vi "clustering.vi"() -> ()   [LabVIEW 2013]
panel:
  in  "sub patterns out":string[](array[string])
  in  "subpatterns out":string[](array[string])
  in  "Sub patterns":string[](array[string])
  in  "top":string[](array[string])=["0 4 0 4 0 4 0 4 0 -2 3 0 3 0 4 0\r\n", "-4 -1\r\n", "-2 0 1 0 -4 4\r\n", "0 4\r\n", "-2 2 0 -1 -4 1 0 3 0\r\n", "-1 0 -1 2\r\n", "0 -1 1 0 4 0 3 -2 0 -2 3 -2 0 4 0 -2 2\r\n", "2 -1 0 4\r\n", "0 4 0 2 0 -2 0\r\n", "1 -1 0 3 0 -4 4 -4 0\r\n", "2 -1 0 3 -2 0 -3 0 3 0 -3 0\r\n", "0 4 0 4 -4 1 -1 0 -3 0 1 -4 1 0 4 0 -4 0 -4 4 -4 1\r\n", "0 -4 1 0 -4 4\r\n", "0 4 0 -2 2 -2 2 -2 2\r\n", "-2 2 -1 0 4 0 2 0 4 0 2 -2 0 4\r\n", "1 0 -1 0 -1 0 1 -1\r\n", "-2 2 -2 3\r\n", "1 0 -1 0 -1 2 0 2 -2 0 -4 0\r\n", "-2 2 0 3 -2 2\r\n", "0\r\n", "1 -1 0 3\r\n", "0 4 0\r\n", "-2 0 1 -4 0 -3 0\r\n", "1 0 -1 2 -1 1 -4\r\n", "0 4\r\n", "-2 0 -1 1\r\n", "0 3 0 3 0 3 -2\r\n", "-4 0 -4 4\r\n", "0 4 0 -4 0 -4\r\n", "-2 2 0 4 -4 0 2 -2\r\n"]
  out "bottom":string[](array[string])
  in  "MOM set 2 bottom CJ vs MOM":string[](array[string])=["-2 0", "0 4 0 3 0 4 0 2 0", "0 3 -2 0 4 0 2 0 4 0 2", "0 2 0 1 0", "0 4 -3 0 -2 0", "0 3 0 4 0 3 0 3 0", "0 3 0 3 0", "0 1 0 -3 3 -3 0 4 0", "0", "0 -3 4 0 3 -2 3 0 1 0 4 0", "0", "0 2 0 3 0 -2 0 -2 0 3 0 1 0", "0 3 0 -3 4 0", "0 3 -2 2 0 3 0 3 0", "0 3 0 3", "0", "-1 0 1", "0 4 0 1", "0 2 0 4 0", "0 1 0 4 0 -4 1 0 3", "0 3", "0 -3 4 0 3 0 3 -2 0 1 0 3 0 3 0", "0 2 0 3", "0 3 0 3 0", "0 1 0 4 0 -2 0 3 0 -4 0 4 0 -4 1 0 3 0 3 0 1", "0 2 0 -3 4 0", "0 3", "0 3", "0 1 0 4", "0", "0 3 0 1 0 3 0 4"]
  in  "WF set 2 bottom CJ vs WF":string[](array[string])=["-2 2 0 4 0 -4 0 3 0", "0 1", "0 3 0 -2 2 -2 3 0 3 -3 0 1 0 3 0 4 0 -2 3", "-2 2 0 3", "0 1 0 4 0 4 -4 1 -1 2 0 3 -3 0 -2", "0 4 -3 0", "0 3", "0 1 0 3 0 2 0 -3 0 4 0 3 0 -2 0 -3 0 -4 0 3 0", "-2 2 -2 3 -3 0 -4 1", "0 4 0", "0 4 0 1 0 4 0 3", "-2 0 2 0 4 0 3", "0 4 0 3 0 4 0 4 0 3 0 3", "-2 2 0 4 0 3 0 2 0 3 -2", "0 3 0 3 0 3 0 3 0 3 0 3 0 4 0 1 0 -2 3 0 3", "0 2 0 -3 4", "1 0 3 0 2", "0 1 0", "-2 2 0 -2 3", "0 1 0 4 0 3 -2 0 -3 0 -3 4 0 1 0 2 0 3 0 1 0 3 0 3 0 4 0 -4 0 3 0 -3 0 2", "0 4 0 1", "0 3 0 4 0 1 0 -2 0", "-2 2 0", "0", "0 2 0", "0 1 0 3", "-2 2 0 -4 4 0 3 0 4 0 -4 0 3 0", "0 2 0 1 0 4 0 1 0 4 0 4 0 3 0", "0 1 0 4 -3 0 2 0 4 0 4 0 -4 0 4 0 1 0 3 0", "0 2 0 3 0"]
  in  "CJ set 2 top CJ vs WF":string[](array[string])=["0 -4 4 -4 0 3 0 4", "0", "-4 1 0 -4 1 0 2 0 -4 0 3 0 1 0 -4 4", "0 -4", "0 2 0 4 -4 0 -1 1 0 -3 0", "-4 0 1", "0 -4 0", "0 -3 0 2 -2 2 0 1 0 1 0 -4 4 -4 1 0 3 0 1", "0 1 0 2", "0 4 -4 1 -4 1 0 1 0 3 0 2", "-4 0 -2 0 2 0 3 0 1", "0 -3 0 4 0 -4 1 -4 1 0", "0 3 0 1 0 3 0 3 0 -4 4 0", "0 4 0 -1 0 3 0 -4 0 1 0 -4 4 -4", "0 -1 1 0 4 -3 4 0 2 0 -4 4 0 -4 4 -4 0 4 0 4 0 1 -1 0 -3 0 -2 3 -2 3 0 3 0 3 0 1 0 -4 0", "0 1 0", "0 3 0 1 0 1 0 4", "0 -3 0 2 -1", "0 4", "0 -3 0 3 0 -4 4 -4 0 -4 4 -4 1 0 2 0 3 0 3 0 4 0 -2 0 1 0 4 0 2 -1 0 3 0 3 0 1", "1 0 4 -4 1 0 2", "0 3 0 2 0 3 0 4 -4 1", "0 4 0 -1 0", "0", "0 4", "-3 0 2 0", "0 -3 0 -3 0 -4 4 0 3 0 2 -2 0 4", "-4 0 4 0 3 0 4 0 3 0 1 0 4", "0 3 0 -4 4 -3 0 4 0 3 0 2 0 2 0 4 0 -4 4 -4 0", "0 1 0 -4 4 -4 0"]
  in  "CJ set 1 bottom CJ vs WF":string[](array[string])=["0 2 0 3 0", "-4 0 4 0 4 0 -4 0 2 0 4", "-1 0 3 0 3 -3 0 4 0 -4 0 3 0", "0 2 0 4 0 3 0 1 0", "0 4 0", "-4 0 3 0 1 0 3", "0 1 0 3 0 1 0 4 0", "0 4 0 3 0 2 0 4 -4 1 0 3 0 3 0 2 0", "0 4", "0 3 0 3 0 3 0 -3 4 0 4 0 2", "-4 1 0 4 -3 0 3 0 4 0 2 0", "0 1 0 4 -3 0 -2 0 -2 2 0 3 0 3 0 -2 2 0 4", "0 1 0 -2 -3 4", "-1 0 4 -3 0 -2 0 1 0 1 0", "0 3", "0 2 -1 0 4 -4 1 0 3 0", "0 1 0 3 0 4 0 3 -2 0", "0 3 0 -4", "0", "0 1 0 -2 0 3 0 1 0 3 0 3 -3 0 4 0", "0 -3 4 0 3 -2 0 -2 2 0 4 0 3 -3 0 1 0 3 0 4 0", "0 3 0 -4 0 2", "0 -4 0 -2 0 -1 0 3 0 1 0 -3 0 3 0 4 0", "-4 0 1 0", "0 4 0", "0 2 0", "0 2 0", "0 3 0 1 0 3 0 -4 0 2 0 -4 0 2 0 -3 4 0 -2 0 3 0 -2 0 -1 1", "0 2 0 4 0 3 -3 4 0 2 0 3 0 1 0 3 0 -4 0 4 0 2 0 4 0 1 0 1 0 2 0 4 -4 1 0 2", "0 1 0 2 0 3 -3 0 1", "-4 0", "0 4 0 -1 0 4", "0 4 0 2 0 4 0 4 -4 0 -2 2 0 -4 4 0 3 0 2 0 2 0 3 0 1 0 2", "0 4", "-1 0 2 0 1"]
  in  "WF set 1 top CJ vs WF":string[](array[string])=["-1 0 1 0", "0 3 0 3 0 3 0 2 0 3 0", "1 0 1 0 4 0 3 0 -2 3 -2 0 3", "0 3 0 1 0 2 0", "0 2 0 4", "0 4 0 1 -1 0 -3", "1 -1 0 4 0 4 0 2 -2 0 -4 0 -3 3 -2 3 0", "2 -1 0 1 0 3 0 3 0 4 0 -4 4 -4 -1 0 3", "0 3", "1 0 2 0 3 0 4 0", "0 2 0 -3 4 0 -1 0 4 0 4 -4 0 2 -1 1 0 3 0", "0 3 -2 3 0 4 0 1 0 4 0 4 0 4 0 3", "2 0 3 0 -4 1 0", "0 1 0 1 -1 0 -1 3 -2 2 0 -3 0 1", "2 0", "0 1 0 3 0 3 0", "0 4 0 1 0 1 0 3 0 4 0 -4 4", "2 0 4 0 -1", "0 3", "0 4 0 1 0 4 -4 0 -3 0 -4 4 0 3 0 -1 1 -4 4", "0 1 0 -4 0 4 0 1 0 4 0 2 0 4 0 2 -2 0 3 0 4 0 3 0 4 0 4", "1 0 4 0 2 0", "2 0 4 0 1 -1 0 4 0 2 0 4 0 1 0 4 0 2", "0 4 0 3 0", "0 3 0 -2 3 0 1", "0 1 0 1 0 -1 0 3 -2 2 0", "2 0 3", "0 1 0 -1 0 2 0 4 0 3 0 1 -1 0 4 -4 0 -1 2 0 1 0 3 0 4 0 3 0 1 -1 0 3", "2 0 3 0 4 0 1 0 4 0 -4 0 3 0 4 0 4 0 2 0 4 0 3 0 3 0 3 -2 3 -3 0 3 0 3 0 -4 1", "1 0 3 0 -3 0 3 0 3 -2 2", "0 4", "2 0 3 0 2 0 -1 0 -3 0", "0 3 0 -4 0 3 0 3 0 3 0 3 0 1 0 3 0 3 0 4 -4 0 1 0 3 0 -3 0 -4 0 3 0 1", "0 -1 0 3", "0 2 0 3 0"]
  in  "CJ set 2 top CJ vs MOM":string[](array[string])=["0 2", "0 2 -1 0 -1 0 4 -4 0 1 0", "-4 1 0 -1 0 -4 4 -4 1 0 4 -4 0", "0 -3 0 2 0", "0 2 0 -4 1 0", "2 0 -2 2 0 -2 0 -4 4 -4 0 4", "0 3 0 -3 4 0 1 0 4", "0 2 0 2 0", "0 4 0", "0 -1 1 -1 0 -2 3 0 1 0 1 0 1 0 3 0", "-4 1 -4 1", "0 -1 0 -4 4 -4 1 -4 1 0 4 -4 1", "0 1 0 1 0 1 0", "0 2 0 -4 0 -1 0 4 -4 0", "-4 1 0 -4 4", "0 3 0 2", "3 0", "0 2 0 -2 0", "-3 0 4 -4 0 4 0", "0 3 0 -2 2 -1 0", "0 -1 0", "0 1 0 1 -4 1 0 4 0 2 0 4 0 3 0 4 -4 1 0 4", "0 4", "-4 1 0 -1 0 -1 0 -2", "-3 0 3 0 -2 0 2 0 4 0 -1 1 0 -2", "-3 0 1 0 1 0", "0 2 -1 0", "1 -4 1 0 4", "0 4 0", "0 2", "0 3 0 4 0 4 -4 0 2"]
  in  "CJ set 1 bottom CJ vs MOM":string[](array[string])=["0 4 -4 0 3 0 4 0", "-4 0 -4 0", "-1 0 3 0 4 0", "0 3", "-1 0 3 0 2 0 4", "-1 0 4 0 2 0 3 -3 0 1 0 2 0", "0 3 -3 0 4", "-1 0 1 0", "2 0 2 0 4 -4 1 0 3", "0 3 0 4 0 -3 0 -3 0 3 -3 0 -2 0 4 0 4 0 -4 0 -4 0 4", "0 -3 0 1 0 4", "0 1 0 -4 0 4 0 -2 0 2 0 4 0 -4 0 3 0 3 0", "-4 0", "0 4 0 -3 0", "-4 4 -4 1 0 -4 4 0 -3 0 -3", "0 -3 3 -3 0 2 0 4 -4 0 -3 3 -3 0", "0 2 0 4 -3 3", "0 -4", "0 2 0 -4 4 0 -2", "-4 1 0 4 0 3 0 3 -2 0 -4 0 1 0 -3 3 -3", "0 -4", "0 -3 0 -3 0 -4 0 -3 3 0", "-1 0 4 0 4 0 4", "0 -3 3 0 2 0 2 0", "0 4 -3 0 4 0 -2 0 4", "-4 0 -4 0 1 -4", "0 4 0 -3 4 0 4", "0 1 0", "0", "-1 0 3 0 3 -3 0 -3 0", "-3"]
  in  "MOM set 1 top CJ vs MOM":string[](array[string])=["2 -1 0 3 0 -2 0 3 0 3", "0 3 -2 2 -1", "1 0 4 0 4 0 2 0 2 0", "2 -1 0", "0 1 0 1 0", "2 0 -2 0 3 -2 0 4", "1 0 4 0 -2 3 -2", "2 0 -2 3", "-3 0 2 0 4 0 4", "-1 0 -1 0 2 0 1 0 4 -4 1 -1 2 -2 3 -2 0 -2 3 0 4 0 3 -2", "2 -1 0 3 -2", "-1 0 2 -2 3 -2 0 -1 0 2 -2 3 0", "0 2", "0 2 0 1", "0 -2 2 -2 3 -2 2 -2 0 1 0", "2 0 2 0 3 -2 2 0 -1 1 0 2", "-1 0 2 -1 0", "2 -2", "-1 0 -1 1 -1 0 -3 0 -2 3 -2", "0 2 -1 0 4 0 -2", "0", "-1 0 2 -1 0 2 -2 3 -2 3 -2 0 2", "2 -2 2 0 2", "-1 0 4 0 3 -2 2 -1 0 -2 3 0 -1", "2 -1 1 -1 0 3 -2 3 0 -2 2 0 -2 3 -2 0 1 0 4 0 2", "0 -2 0 2 -2", "-1 0 2 0 2 0 -2 3", "2 0", "0 -1 0 -2 0 -2", "-1 0", "-1"]
  in  "HY set 2 bottom CJ vs HY":string[](array[string])=["0 2 0", "0 4", "0 1 0", "0", "0 3 0 3 0 -1 0 4 0 -3", "0 4 0 -2 0 1 0 4 0 4 0 1 0 3 -3 0", "0 1 0 2", "0 2 0 4", "1 0 1 0 3 0 3 0 3", "0 1 0 4 0 3 0 -2 0", "-1 0 2 0 3 0 -4 1 0 4 0", "0 2 0 -4 0 -4 4 0", "0 1 -1 2", "0 4 0 2 0 3 0 -2 0 -4", "0", "0 1", "0 4 0 -1 1 0", "0", "0", "0 1 0 4 0 -4 0 4 0 -4 0", "0 3 0 -2 0 3 0 2", "0 1", "0 2", "0", "-1 0 4 0 -3 0 -2 0 -2 0 1 0 -4 0 4", "2 -1", "0 -1 0 4 0 4 -4 0 -1 2", "0 -2 0", "0 3 0", "-1 0 -3 0", "0 2 0 1", "0 1 0 1", "0 4 0 2 0 -4 1 2 0 4 0 4 0 4", "0"]
  in  "CJ set 2 top CJ vs HY":string[](array[string])=["0 -1 1", "0 1 0", "0 3 0 4 0 -1 0", "0 4 -4 0 1", "0 4 0 1 -1 0 -3 0 4 0 -1 0 4", "0 -3 0 2 0 4 0 2 -1 0 4 -4", "0 1", "0 4 0 1 0 -1 0", "0 2 -1 0 -4 4 0 1", "0 2 0 4 -4 1", "4 -4 0 4 0 2 0 3 0 4", "0 4 0 2 0 4", "0 -1 1 -1", "0 -4 0 -4 4 0 4 0 4 -4 1 0 3", "0 -1", "0 2 0 2", "0 3 0 1 0", "0 2 0", "0", "0 4 -4 1 -4 0 3 -2 0 4 0 4 0", "0 2 0 4 -4 1 0 1", "0", "0", "0", "0 2 0 -1 0 4 -4 1 0 1 0 1 0 4 0 4 0 2", "0 -1", "-4 1 0 4 0 -2 0 3 0 -1 1", "0 -2 0 -4 0 4 -3 0", "0 -1 1 0", "4 0", "0 4 0", "0", "0 -4 0 4 0 2 -1 1 0 4 0 -3 0 -4 0 2 0 3 0 2 0", "0"]
  in  "CJ set 1 bottom CJ vs HY":string[](array[string])=["2 0 3 0 3 0 4 0 4 0 3", "0", "0 4 -3 0 3 0", "-1 0 4 1 0 3", "-4", "0 3 0 2 0", "0 1", "0 -3 3 0 3 -3 0 4 0 1 0 3 0 1", "-1 0 -1 0", "-4 0 -4 0 4 -4 0", "-1 0 4 0 2 0 3 0", "-1 0 1 0 3 -3 0 1 0", "0 2 0 3 0 2 0 4 0 4 0 2 0 3 0 2", "0 3", "1 -4 0", "0 -1 0 1 -4 4 0 3 0 4 0 2 0", "0 4 0 -2 2 0", "0 4", "0 1 0 4 0 3 0 3", "0 1 0", "0 2 0", "-1 0 4", "-4 0 -2 3", "0 3 0 1 0", "-1 0 1 -1", "0 2 0 3 0", "0 4 0", "-4 0 -4 0 4 0", "0 3 0", "0 3", "0 1 0"]
  in  "HY set 1 top CJ vs HY":string[](array[string])=["0 4 0 4 0 3 0 -2 3 0 4 0", "1", "2 -2 0 4", "1 0 4", "0", "-2 0 1 -4 1 0 3", "1 0", "0 -1 1 0 -4 0 3 0 3 0 4 0 -2 2", "2 0 4", "0 2 0 -2 0", "1 -1 0 3 0 4 -4 4 0", "0 3 2 0 -3 0 3 0 4", "0 -4 4 0 1 0 -3 0 1 0 4 0 -4 4 -4", "1 0 -4 4", "-3 0 4 0 2", "-2 2 0 4 0 2 0 4 0 2 0 -4 0", "1 0 -1 0 -1 0 1", "2 0 3", "1 0 2 0 3 0 2 0 -4 0", "-2 2 0 3 -2", "0", "1 -1 0 3", "0", "-2 0 1 0", "0 -1 2 -1 1", "0 4", "2 0 -1", "0 3 0 3 0 3", "0", "0 4 0", "2 0 2"]
  in  "CJ set 2 bottom CJ vs DU":string[](array[string])=["0 1 0 3", "0 2 0 3 0 3 -2 2 0 4 -4 1 0 4 0 2 0 4 0 4 0 2 0", "0 -3 3 0 -2", "1 0 1 0 -2 0 1 0 -2 2 0", "0 3", "1 0 3 0 2 0 3 0", "0 4 0 1 0", "0 2", "1", "0 2 0 -3 4 0 4", "0 2 0 3 0", "0", "0 2 0 3 0 1 0 -2 2 0 3 0", "0 1 0 4 -4", "0 -3 0 -2 2 -2 3 -2 2 -2", "0 2 0", "0 3 -2 0", "0 3", "0 3 0 3", "0 1 0", "0 2 0 3 0 4 0 2 0", "0 4 0 4 -3", "0 1 0 -3", "0 4 0 1 0", "0 3 0 -2", "0 2 0 3 -2 2 0 -2 0 -3 4 0", "0 1 0 3 0", "-1 0 3", "0 3 0 2 0 3", "0 2 0 4", "0 4 0 2 0 4 -4", "1 0 3 0 3 -2 2 0 4 0 3 0 1 0 -2", "0 -3 4 -3", "2 0 2 0 3 -3 0", "0 1 0 3 0 1 0 4", "0 1 0", "-1 0 1 0", "0 3 -3 0 1 0", "0 2 0 3 0 -2"]
  in  "DU set 2 top CJ vs DU":string[](array[string])=["0 2 0 4 -4 1", "-4 1 0 2 0 2 0 -2 0 -4 4 -4 1 0 3 0 4", "0 1 -4 1 0 4 -4", "-3 0 3 0 -4 0 1 -4", "0 1 0", "0 3 -2 0 1 0 -4 4 0 2 0", "-4 0 2 0 4", "0", "0", "0 1 0", "0 -4 0 3 0 2 0 4 0 4 0 -1 0 -4 0 -2 0", "1 0 4", "0 4 0 -1 0 2 0 4 -4 1 0 4 0", "0 4 0 2 0", "-4 0 1 0 1 0 1 0 -4", "0 -4", "0 4 0 2 0", "-4 1 0", "0 -1 0", "0 3 0", "0 -4 4 0 4 0 2 0 1 -4", "1 0 1", "-1 0 -1 0 2 0 2", "-4 -1 0", "0 1 0 4 0 4", "0 3 0 1 0 1", "0 4 -4 1 0", "0 1 0 4", "0 2 0 -2 0 1 -4", "0", "0 2 0 1 -4 4 0 2", "0 4 0 1 0 1 0 1 0 2 0 4 0 4 -4 1", "-4 1 0 1 0 4", "0 -3 0 -4 0 -2", "0 4 0 2", "-1 0 -1 0 4 0", "-4 1 0 -1 2 0 4", "0 2 0", "0 1 0 -4 0 -4 4 -4 1"]
  in  "DU set 1 bottom CJ vs DU":string[](array[string])=["0 3 -3 4 0 4 0", "0 3", "0 4 0 1 0 4 0", "0", "0 3 0 1 0 3 -3 0 4 0 -2 3", "0 3 0 1", "0 1 0 3", "0 3 0 -3", "0", "0 -3 4 0 2 0 -3 0 3 0 3 -3 0 4", "0 -1 0 4 0 1", "0", "-1 0 3", "0 4 -3 0 3 0 -3 4 -3 0 3 -2 2 0 -3 0", "0 2 0 1 0 3 0 4 0 2 0 4 0 -3 4 -3 0", "0 4", "0 -2 0 3", "0 3 0 3", "-1 0 -1 0 4 0 2 0 4 0 -2 0 4 0 2 0 3 0", "0 4 0 1 0 3 0 4 0 4 -4 1 0", "0", "0 -3", "0 3 0 1 0 3", "0", "0 1 0", "0 3 0", "0 1 0 4", "-1 0 1 0 3", "0 -3", "0 3", "0", "0 -2 0 -4 0", "0 4 0 3 0 4 0"]
  in  "CJ set 1 top CJ vs DU":string[](array[string])=["0 -3 0 1 0 -3 3 0 -3 0", "-1 4 -4 1 0", "0 2 0 -1 0 -3 3", "0 4", "0 3 0 -4 4 -4", "0 -4 0 -2 0 1", "-4 1 0 1 0", "0 -1 0 4 0 1 0", "0", "0 -1 0 -4 1 0 -4 0 2 0", "-1 -4 1 0 -1 0", "0 1 0 3", "3 -1 3 0 2 0 -4", "0 4 0 -3 0 1 0 1 0 4 -4 0 3", "0 4 0 2 0 3 0 3 0 -4 1 0 -3 0 3 -2 3", "0 3 0", "0 4 0 1 0 -4 4", "0 4 0", "-1 -4 1 -1 0 4 0 2 0 -4 1 -4 0 -3 0 -3 0 -4 0 -1 0 4", "2 0 2 0 4 -4 4 -4 1 0 1 0 4 0 1 -4 0 3", "0", "0", "0 4 0 -4 0 4 0", "1", "0 4", "0 1 0 4 0", "0 2 -2 0 -3 0 3 0", "-1 4 -4 1 0 4", "0 3 0 1 0", "0 4 -4 0", "0", "-1 0 4 0 4 0 3", "0 3 0 1 0 4 0 -3 0 -4"]
  in  "movement sequences":string[](array[string])=["0 4 0 4 0 4 0 4 0 3 0 -2 3 0 4 0\r\n", "4 -4 0 -1\r\n", "0 4\r\n", "2 -2 0 1 -4 1 0 1 0 -3 3\r\n", "0 -1\r\n", "0 1 0 -4 0 3 0 3 0 4 0 2 0 2\r\n", "2 0 4\r\n", "0 4 0 4 0\r\n", "0 -1 0 3 0 -4 0 4 0\r\n", "2 0 2 0 3 0 4 0\r\n", "0 -4 0 1 0 4 0 1 -4 0 4 0 4 -4\r\n", "1 0 4\r\n", "0 2\r\n", "2 -2 2 -1 0 4 0 2 0 4 0 2 0 -4 0\r\n", "0 1 0 -1 0 1\r\n", "0 3\r\n", "0 -1 0 2 0 2 -2 0 -4 0\r\n", "1 0 2 0 3 -2\r\n", "-2 0\r\n", "0 -1 0 -1 0 3\r\n", "0 4 0\r\n", "0 1 0 -3\r\n", "0 -1 1 -4\r\n", "0 4\r\n", "0 -1 1\r\n", "0 3 0 -3 0 3\r\n", "0\r\n", "0 -4 4 0 -4 0 -4\r\n", "2 0\r\n"]
  out "4":string[](array[string])
  out "3":string[](array[string])
  out "2":string[](array[string])
  out "1":string[](array[string])
  out "0":string[](array[string])
  out "Cluster":dbl[](array[numeric])
  out "weighted score cluster 4":dbl[](array[numeric])
  out "weighted score cluster 3":dbl[](array[numeric])
  out "weighted score cluster 2":dbl[](array[numeric])
  out "Transition number":i32[](array[numeric])
  out "weighted score cluster 1":dbl[](array[numeric])
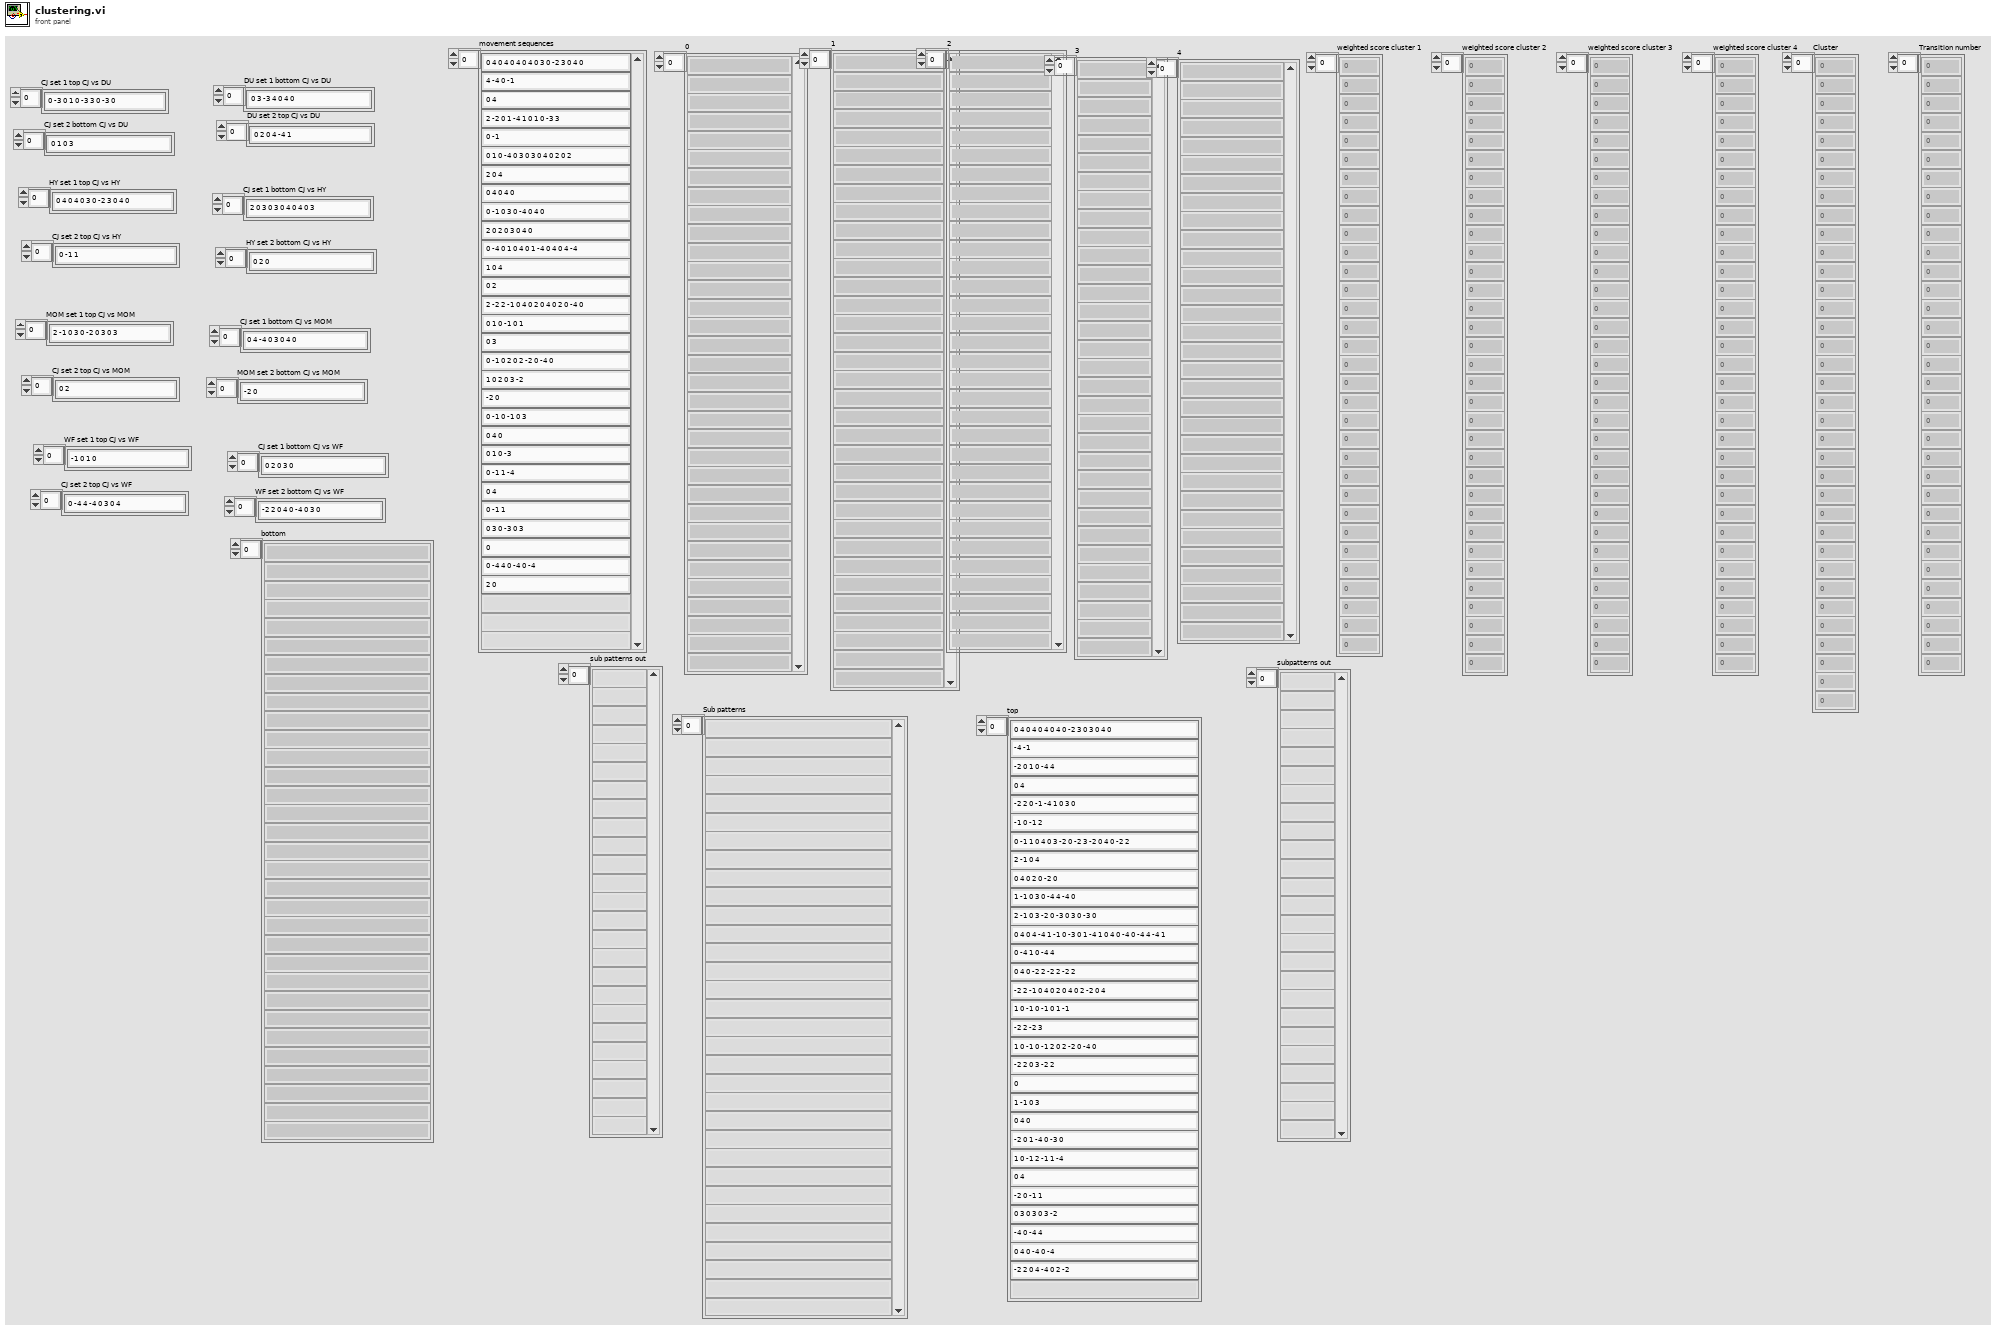
[diagram p1: front panel]
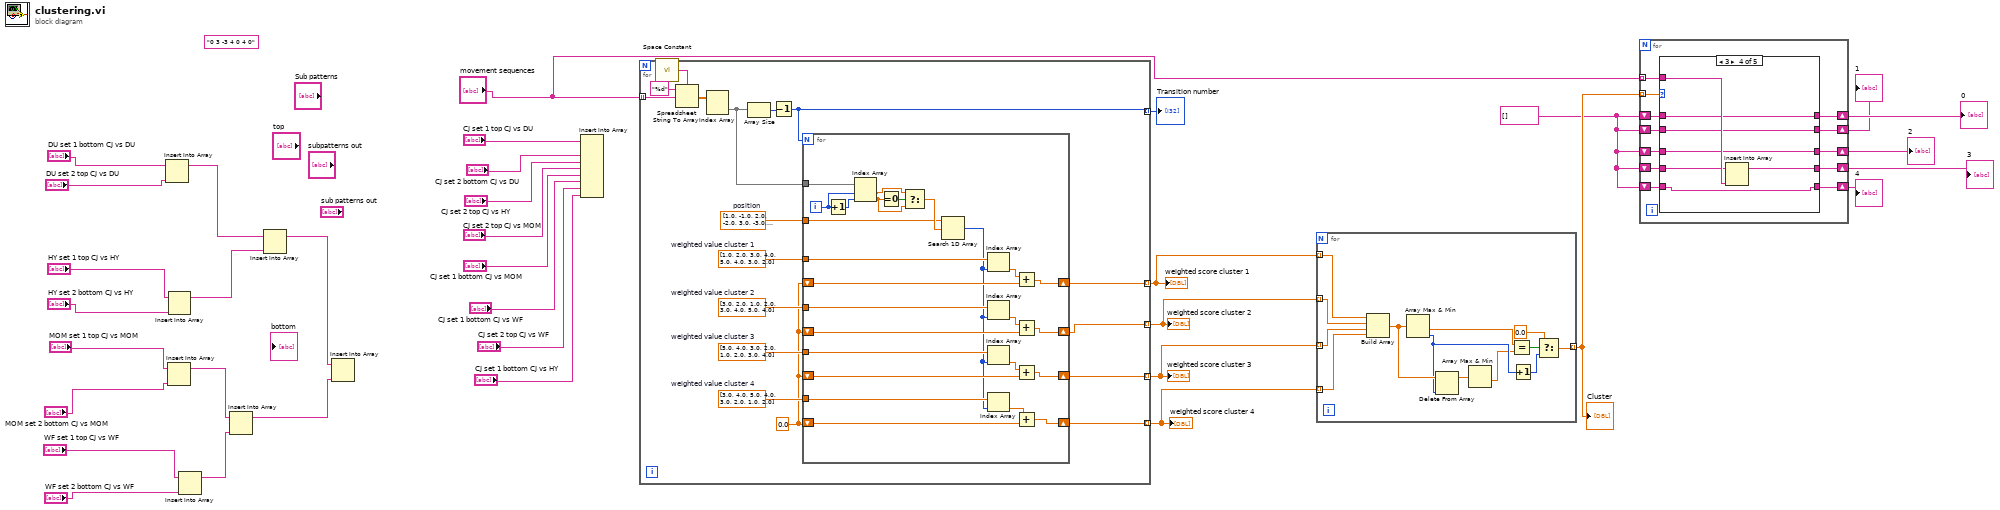
[diagram p0: block diagram]
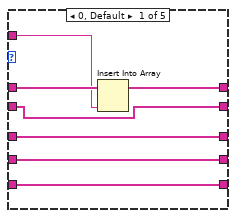
[diagram p2: hidden frame]
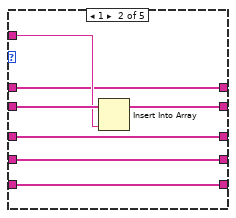
[diagram p3: hidden frame]
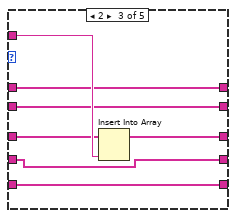
[diagram p4: hidden frame]
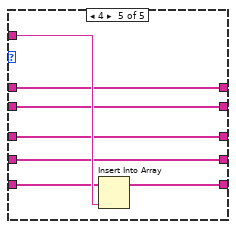
[diagram p5: hidden frame]
diagram:
  (unwired) "0 3 -3 4 0 4 0" ("String")
  w29 = string[] [] ("movement sequences")
  n1 = Insert Into Array(array="DU set 1 bottom CJ vs DU", new element="DU set 2 top CJ vs DU") -> (w8:string[])  [unwired: 1 in]
  n2 = Insert Into Array(array="MOM set 1 top CJ vs MOM", new element="MOM set 2 bottom CJ vs MOM") -> (w6:string[])  [unwired: 1 in]
  n3 = Insert Into Array(array="HY set 1 top CJ vs HY", new element="HY set 2 bottom CJ vs HY") -> (w7:string[])  [unwired: 1 in]
  n4 = Insert Into Array(array="WF set 1 top CJ vs WF", new element="WF set 2 bottom CJ vs WF") -> (w5:string[])  [unwired: 1 in]
  n5 = Insert Into Array(array=w6, new element=w5) -> (w4:string[])  [unwired: 1 in]
  n6 = Insert Into Array(array=w8, new element=w7) -> (w3:string[])  [unwired: 1 in]
  n7 = Insert Into Array(array=w3, new element=w4) -> ()  [unwired: 1 in, 1 out]
  n8 = Insert Into Array(array="CJ set 1 top CJ vs DU", new element #1="CJ set 2 bottom CJ vs DU", new element #2="CJ set 2 top CJ vs HY", new element #3="CJ set 2 top CJ vs MOM", new element #4="CJ set 1 bottom CJ vs MOM", new element #5="CJ set 1 bottom CJ vs WF", new element #6="CJ set 2 top CJ vs WF", new element #7="CJ set 1 bottom CJ vs HY") -> ()  [unwired: 1 in, 1 out]
  n9 = for {
    tunnel: "movement sequences" -> [w52] mode=indexing
    tunnel: [w46] -> w34 mode=indexing
    tunnel: [w39] -> w35 mode=indexing
    tunnel: [w38] -> w33 mode=indexing
    tunnel: [w37] -> w32 mode=indexing
    tunnel: [w36] -> w31 mode=indexing
    w42 = dbl[] [5.0, 4.0, 3.0, 2.0, 1.0, 2.0, 3.0, 4.0]  # weighted value cluster 3
    w43 = dbl[] [3.0, 2.0, 1.0, 2.0, 3.0, 4.0, 5.0, 4.0]  # weighted value cluster 2
    w44 = dbl[] [1.0, 2.0, 3.0, 4.0, 5.0, 4.0, 3.0, 2.0]  # weighted value cluster 1
    w41 = dbl[] [3.0, 4.0, 5.0, 4.0, 3.0, 2.0, 1.0, 2.0]  # weighted value cluster 4
    w45 = dbl[] [1.0, -1.0, 2.0, -2.0, 3.0, -3.0, 4.0, -4.0]  # position
    w40 = 0.0
    n10 = call <vilib>:"Space Constant.vi"() -> ("String"=w50:string)
    n11 = Spreadsheet String To Array(delimiter (Tab)=w50, format string="%d", spreadsheet string=w52) -> (array=w49:dbl[][])  [unwired: 1 in]
    n12 = Index Array(array=w49) -> (element=w47:dbl[])  [unwired: 2 in]
    n13 = Array Size(array=w47) -> (size(s)=w48:i32)
    n14 = Decrement(x=w48) -> (x-1=w39:i32)
    n15 = for {
      N: w39 -> [_]
      tunnel: w47 -> [w77]
      shift-right: [w69] -> w46
      shift-left: w40 -> [w68]
      tunnel: w45 -> [w67]
      tunnel: w44 -> [w66]
      shift-right: [w57] -> w38
      shift-left: w40 -> [w54]
      shift-right: [w58] -> w37
      shift-left: w40 -> [w55]
      shift-right: [w59] -> w36
      shift-left: w40 -> [w56]
      tunnel: w43 -> [w62]
      tunnel: w42 -> [w61]
      tunnel: w41 -> [w60]
      i -> [w76]
      n16 = Increment(x=w76) -> (x+1=w75:i32)
      n17 = Index Array(array=w77, index #1=w76, index #2=w75) -> (element #1=w73:dbl, element #2=w72:dbl)
      n18 = Equal To 0?(x=w72) -> (x = 0?=w74:bool)
      n19 = Select(t=w73, s=w74, f=w72) -> (s? t:f=w71:dbl)
      n20 = Search 1D Array(1D array=w67, element=w71) -> (index of element=w53:i32)  [unwired: 1 in]
      n21 = Index Array(array=w66, index=w53) -> (element=w70:dbl)
      n22 = Index Array(array=w62, index=w53) -> (element=w65:dbl)
      n23 = Index Array(array=w61, index=w53) -> (element=w64:dbl)
      n24 = Index Array(array=w60, index=w53) -> (element=w63:dbl)
      n25 = Add(x=w70, y=w68) -> (x+y=w69:dbl)
      n26 = Add(x=w65, y=w54) -> (x+y=w57:dbl)
      n27 = Add(x=w64, y=w55) -> (x+y=w58:dbl)
      n28 = Add(x=w63, y=w56) -> (x+y=w59:dbl)
    }
  }
  "weighted score cluster 1" <- w34
  "Transition number" <- w35
  "weighted score cluster 2" <- w33
  "weighted score cluster 3" <- w32
  "weighted score cluster 4" <- w31
  n29 = for {
    tunnel: w34 -> [w90] mode=indexing
    tunnel: w33 -> [w89] mode=indexing
    tunnel: w32 -> [w88] mode=indexing
    tunnel: w31 -> [w87] mode=indexing
    tunnel: [w80] -> w30 mode=indexing
    n30 = Build Array(w90, w89, w88, w87) -> (w86:dbl[])
    n31 = Array Max & Min(array=w86) -> (min value=w78:dbl, min index (indices)=w82:i32)  [unwired: 2 out]
    n32 = Delete From Array(array=w86, index=w82) -> (array with subset deleted=w85:dbl[])  [unwired: 1 in, 1 out]
    n33 = Array Max & Min(array=w85) -> (min value=w79:dbl)  [unwired: 3 out]
    n34 = Equal?(x=w78, y=w79) -> (x = y?=w84:bool)
    n35 = Increment(x=w82) -> (x+1=w81:i32)
    n36 = Select(t=0.0, s=w84, f=w81) -> (s? t:f=w80:dbl)
  }
  "Cluster" <- w30
  n37 = for {
    tunnel: w30 -> [w102] mode=indexing
    tunnel: "movement sequences" -> [w101] mode=indexing
    shift-right: [w99] -> w28
    shift-left: w29 -> [w100]
    shift-right: [w97] -> w27
    shift-left: w29 -> [w98]
    shift-right: [w95] -> w26
    shift-left: w29 -> [w96]
    shift-right: [w93] -> w25
    shift-left: w29 -> [w94]
    shift-right: [w91] -> w24
    shift-left: w29 -> [w92]
    n38 = case shown="3" w102 {
      tunnel: w101 -> [w107 w114 w123 w130 w137]
      tunnel: w100 -> [w109 w113 w120 w127 w131]
      tunnel: [w108 w113 w120 w127 w131] -> w99
      tunnel: w98 -> [w106 w116 w119 w126 w132]
      tunnel: [w106 w115 w119 w126 w132] -> w97
      tunnel: w96 -> [w105 w112 w122 w125 w133]
      tunnel: [w105 w112 w121 w125 w133] -> w95
      tunnel: w94 -> [w104 w111 w118 w129 w134]
      tunnel: [w104 w111 w118 w128 w134] -> w93
      tunnel: w92 -> [w103 w110 w117 w124 w136]
      tunnel: [w103 w110 w117 w124 w135] -> w91
      frame 0, Default {
        n39 = Insert Into Array(array=w109, new element=w107) -> (w108:string[])  [unwired: 1 in]
      }
      frame 1 {
        n40 = Insert Into Array(array=w116, new element=w114) -> (w115:string[])  [unwired: 1 in]
      }
      frame 2 {
        n41 = Insert Into Array(array=w122, new element=w123) -> (w121:string[])  [unwired: 1 in]
      }
      frame 3 {
        n42 = Insert Into Array(array=w129, new element=w130) -> (w128:string[])  [unwired: 1 in]
      }
      frame 4 {
        n43 = Insert Into Array(array=w136, new element=w137) -> (w135:string[])  [unwired: 1 in]
      }
    }
  }
  "0" <- w28
  "1" <- w27
  "2" <- w26
  "3" <- w25
  "4" <- w24
